vi "Ponit_Size.vi"(0 "New Value":dbl format="%.2f", 1 "Array In":dbl[][](array[numeric]) format="%.2f", 2 "Index1":i32, 3 "Index2":i32, 4 "Size":i32) -> (5 "Array Out":dbl[][](array[numeric]) format="%.2f")   [LabVIEW 2010]
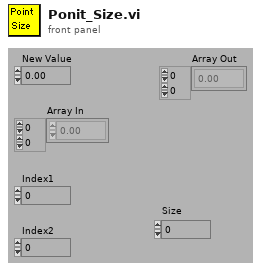
[diagram p1: front panel]
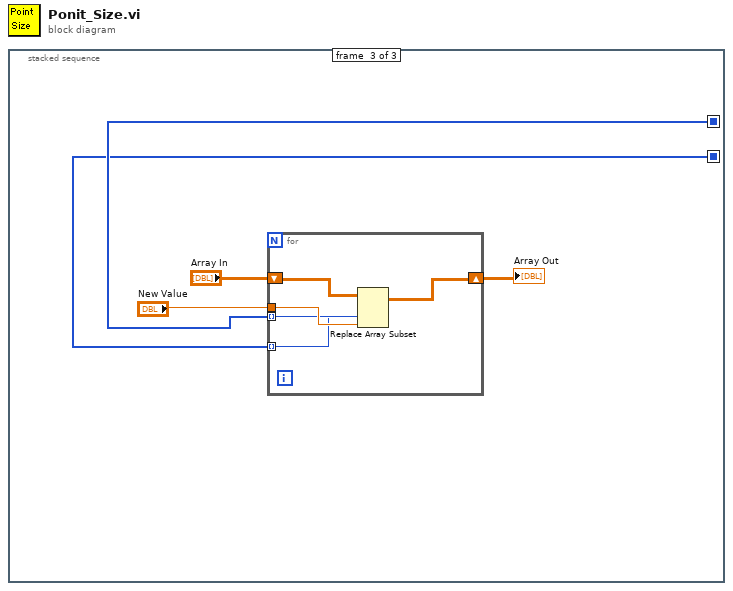
[diagram p0: block diagram]
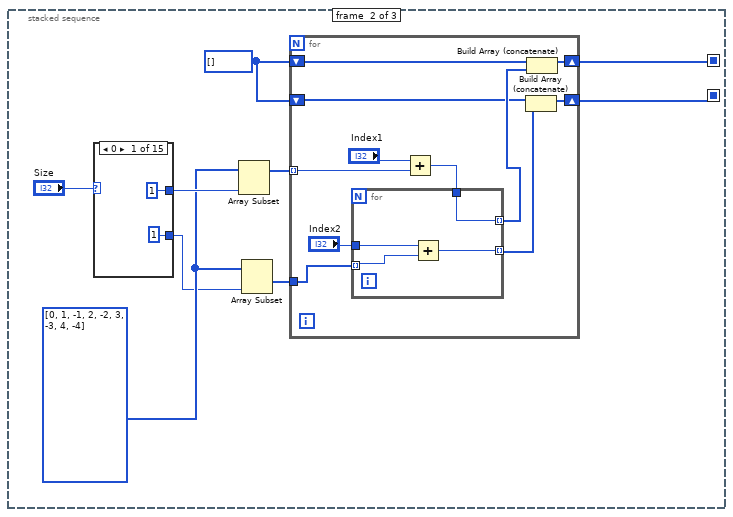
[diagram p3: hidden frame]
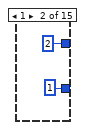
[diagram p4: hidden frame]
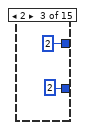
[diagram p5: hidden frame]
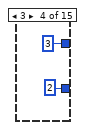
[diagram p6: hidden frame]
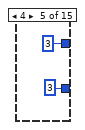
[diagram p7: hidden frame]
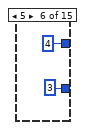
[diagram p8: hidden frame]
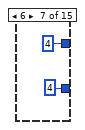
[diagram p9: hidden frame]
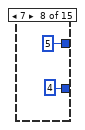
[diagram p10: hidden frame]
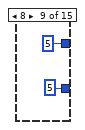
[diagram p11: hidden frame]
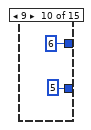
[diagram p12: hidden frame]
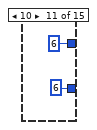
[diagram p13: hidden frame]
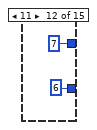
[diagram p14: hidden frame]
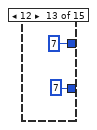
[diagram p15: hidden frame]
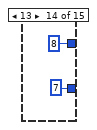
[diagram p16: hidden frame]
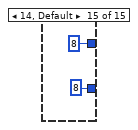
[diagram p17: hidden frame]
diagram:
  n1 = stacked-sequence {
    seq-local: [_ w8 _] -> [_ _ w56]
    seq-local: [_ w7 _] -> [_ _ w55]
    frame #0 {
    }
    frame #1 {
      w3 = i32[] [0, 1, -1, 2, -2, 3, -3, 4, -4]
      w9 = i32[] []
      n2 = case shown="0" "Size" {
        tunnel: [1 2 2 3 3 4 4 5 5 6 6 7 7 8 8] -> w4
        tunnel: [1 1 2 2 3 3 4 4 5 5 6 6 7 7 8] -> w2
        frame 0 {
        }
        frame 1 {
        }
        frame 2 {
        }
        frame 3 {
        }
        frame 4 {
        }
        frame 5 {
        }
        frame 6 {
        }
        frame 7 {
        }
        frame 8 {
        }
        frame 9 {
        }
        frame 10 {
        }
        frame 11 {
        }
        frame 12 {
        }
        frame 13 {
        }
        frame 14, Default {
        }
      }
      n3 = Array Subset(array=w3, length=w4) -> (w5:i32[])  [unwired: 1 in]
      n4 = Array Subset(array=w3, length=w2) -> (w1:i32[])  [unwired: 1 in]
      n5 = for {
        tunnel: w5 -> [w50] mode=indexing
        shift-right: [w46] -> w8
        shift-left: w9 -> [w47]
        shift-right: [w44] -> w7
        shift-left: w9 -> [w45]
        tunnel: w1 -> [w40]
        n6 = Add(x="Index1", y=w50) -> (x+y=w49:i32)
        n7 = for {
          tunnel: "Index2" -> [w54]
          tunnel: [w53] -> w43 mode=indexing
          tunnel: [w52] -> w48 mode=indexing
          tunnel: w49 -> [w52]
          tunnel: w40 -> [w51] mode=indexing
          n8 = Add(x=w54, y=w51) -> (x+y=w53:i32)
        }
        n9 = Build Array (concatenate)(w45, w43) -> (w44:i32[])
        n10 = Build Array (concatenate)(w47, w48) -> (w46:i32[])
      }
    }
    frame #2 {
      n11 = for {
        tunnel: "New Value" -> [w64]
        shift-right: [w63] -> w59
        shift-left: "Array In" -> [w62]
        tunnel: w56 -> [w61] mode=indexing
        tunnel: w55 -> [w60] mode=indexing
        n12 = Replace Array Subset(array=w62, new element=w64, index (row)=w61, index (col)=w60) -> (w63:dbl[][])
      }
      "Array Out" <- w59
    }
  }
